vi "Stirling's Formula.vi"(3 "x":dbl format="%.2f") -> (1 "Stirling(x)":dbl format="%.2f")   [LabVIEW 2020, in "NI_Gmath.lvlib"]
doc: "Computes the Stirling approximation to the gamma function."
uses:
  <vilib>/gmath/NI_Gmath.lvlib
  <resource>/lvanlys.dll
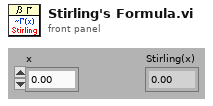
[diagram p1: front panel]
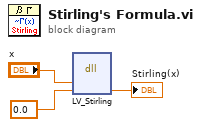
[diagram p0: block diagram]
diagram:
  n1 = dll-call lib="e:/builds/penguin/labview/branches/2020/dev/dist/resource/lvanlys.*" fn="LV_Stirling"("x"="x", "Stirling(x)"=0.0 ("Stirling")) -> ("Stirling(x)"=→"Stirling(x)":dbl)  [unwired: 5 in, 2 out]
